vi "associate mirrors and cameras.vi"(1 "Mirrors":u8[](array[numeric]), 2 "DeviceList":T3(array[cluster])) -> (0 "CamConfigArray":T2(array[cluster]))   [LabVIEW 2013]
uses:
  <vilib>/userdefined/High Color/IMAQdx.ctl
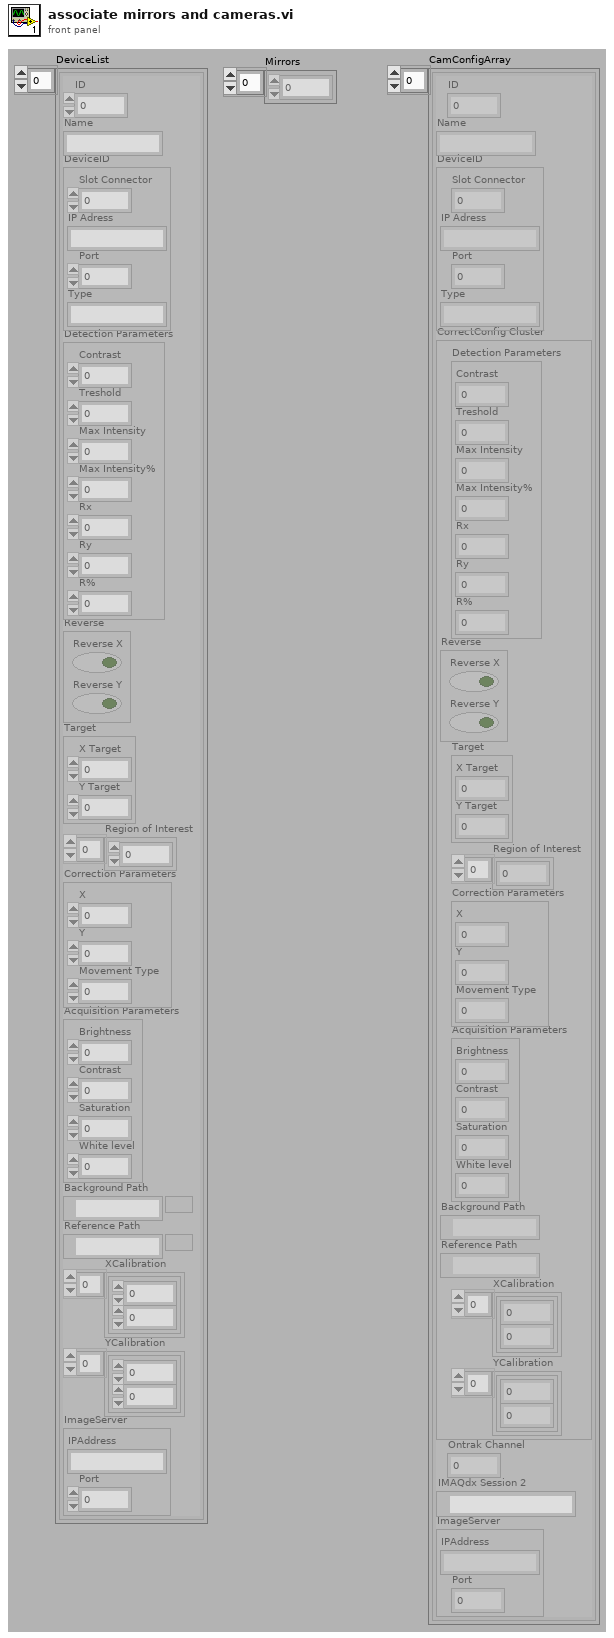
[diagram p1: front panel]
types:
  T1 = typedef "IMAQdx.ctl" = refnum<k21>
  T2 = cluster{"ID":dbl, "Name":string, "DeviceID":cluster{"Slot Connector":i32, "IP Adress":string, "Port":i32, "Type":string}, "CorrectConfig Cluster":cluster{"Detection Parameters":cluster{"Contrast":i32, "Treshold":u8, "Max Intensity":i32, "Max Intensity%":u8, "Rx":i32, "Ry":i32, "R%":sgl}, "Reverse":cluster{"Reverse X":bool, "Reverse Y":bool}, "Target":cluster{"X Target":sgl, "Y Target":sgl}, "Region of Interest":i32[], "Correction Parameters":cluster{"X":sgl, "Y":sgl, "Movement Type":u16}, "Acquisition Parameters":cluster{"Brightness":dbl, "Contrast":dbl, "Saturation":dbl, "White level":dbl}, "Background Path":path, "Reference Path":path, "XCalibration":cluster{dbl, dbl}[], "YCalibration":cluster{dbl, dbl}[]}, "Ontrak Channel":i16, "IMAQdx Session 2":T1, "ImageServer":cluster{"IPAddress":string, "Port":i32}}[]
  T3 = cluster{"ID":dbl, "Name":string, "DeviceID":cluster{"Slot Connector":i32, "IP Adress":string, "Port":i32, "Type":string}, "Detection Parameters":cluster{"Contrast":i32, "Treshold":u8, "Max Intensity":i32, "Max Intensity%":u8, "Rx":i32, "Ry":i32, "R%":sgl}, "Reverse":cluster{"Reverse X":bool, "Reverse Y":bool}, "Target":cluster{"X Target":sgl, "Y Target":sgl}, "Region of Interest":i32[], "Correction Parameters":cluster{"X":sgl, "Y":sgl, "Movement Type":u16}, "Acquisition Parameters":cluster{"Brightness":dbl, "Contrast":dbl, "Saturation":dbl, "White level":dbl}, "Background Path":path, "Reference Path":path, "XCalibration":cluster{dbl, dbl}[], "YCalibration":cluster{dbl, dbl}[], "ImageServer":cluster{"IPAddress":string, "Port":i32}}[]
  T4 = cluster{"Detection Parameters":cluster{"Contrast":i32, "Treshold":u8, "Max Intensity":i32, "Max Intensity%":u8, "Rx":i32, "Ry":i32, "R%":sgl}, "Reverse":cluster{"Reverse X":bool, "Reverse Y":bool}, "Target":cluster{"X Target":sgl, "Y Target":sgl}, "Region of Interest":i32[], "Correction Parameters":cluster{"X":sgl, "Y":sgl, "Movement Type":u16}, "Acquisition Parameters":cluster{"Brightness":dbl, "Contrast":dbl, "Saturation":dbl, "White level":dbl}, "Background Path":path, "Reference Path":path, "XCalibration":cluster{dbl, dbl}[], "YCalibration":cluster{dbl, dbl}[]}
  T5 = cluster{"Slot Connector":i32, "IP Adress":string, "Port":i32, "Type":string}
  T6 = cluster{"ID":i32, "Name":string, "DeviceID":cluster{"Slot Connector":i32, "IP Adress":string, "Port":i32, "Type":string}, "CorrectConfig Cluster":cluster{"Detection Parameters":cluster{"Contrast":i32, "Treshold":u8, "Max Intensity":i32, "Max Intensity%":u8, "Rx":i32, "Ry":i32, "R%":sgl}, "Reverse":cluster{"Reverse X":bool, "Reverse Y":bool}, "Target":cluster{"X Target":sgl, "Y Target":sgl}, "Region of Interest":i32[], "Correction Parameters":cluster{"X":sgl, "Y":sgl, "Movement Type":u16}, "Acquisition Parameters":cluster{"Brightness":dbl, "Contrast":dbl, "Saturation":dbl, "White level":dbl}, "Background Path":path, "Reference Path":path, "XCalibration":cluster{dbl, dbl}[], "YCalibration":cluster{dbl, dbl}[]}, "Ontrak Channel":i16, "IMAQdx Session 2":T1, "ImageServer":cluster{"IPAddress":string, "Port":i32}}
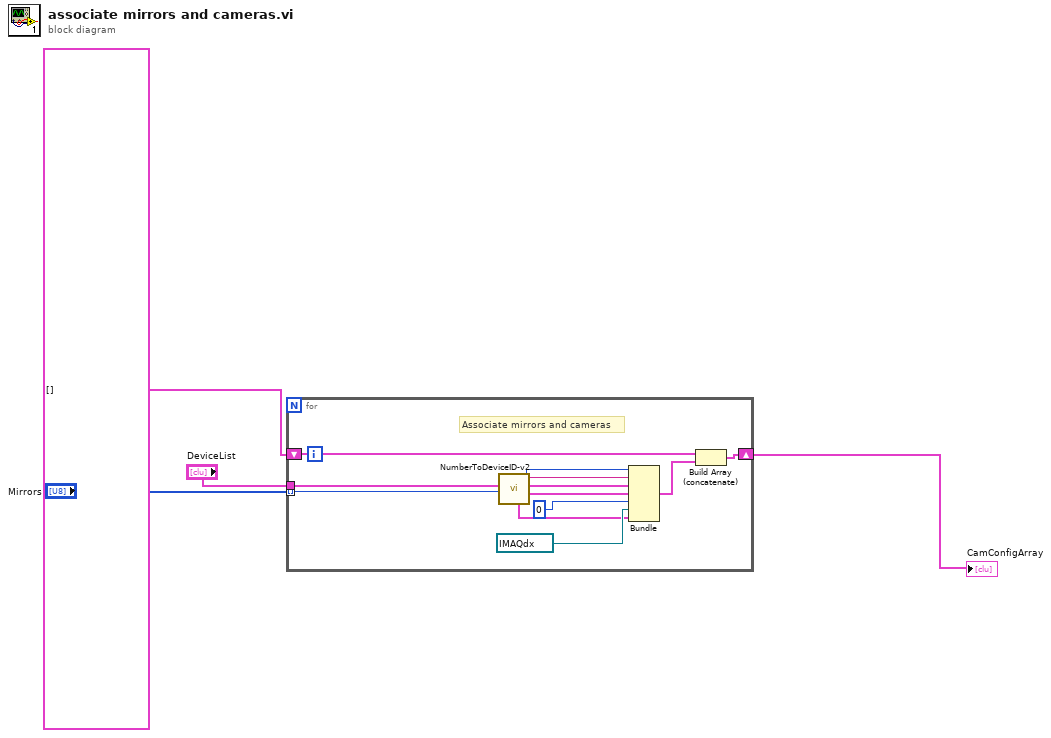
[diagram p0: block diagram]
diagram:
  n1 = for {
    shift-right: [w15] -> w3
    shift-left: T2 [] ("CamConfigArray 2") -> [w16]
    tunnel: "Mirrors" -> [w12] mode=indexing
    tunnel: "DeviceList" -> [w5]
    # "Associate mirrors and cameras"
    n2 = call "NumberToDeviceID-v2.vi"("device raw"=w12, "DeviceList"=w5) -> ("ID"=w10:i32, "CorrectConfig Cluster"=w9:T4, "DeviceID"=w13:T5, "Name"=w14:string, "ImageServer"=w6:cluster{"IPAddress":string, "Port":i32})  [unwired: 5 in]
    n3 = Bundle("ID"=w10, "Name"=w14, "DeviceID"=w13, "CorrectConfig Cluster"=w9, "Ontrak Channel"=i16 0, "IMAQdx Session 2"=T1 "cam2", "ImageServer"=w6) -> (w11:T6)  [unwired: 1 out]
    n4 = Build Array (concatenate)(w16, w11) -> (w15:T2)
  }
  "CamConfigArray" <- w3
